vi "例程11-全局.vi"() -> ()   [LabVIEW 2016]
panel:
  in  "开关":bool
  in  "数值":i32
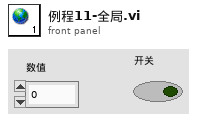
[diagram p1: front panel]
diagram:
